vi "HTTP_Post.vi"(4 "data":string, 5 "URL":string="http://localhost:8086/api/v2/write?org=hassiosp&bucket=hassiosp&precision=ns", 6 "error in (no error)":errorcluster, 7 "value 3":string="application/json", 8 "value 2":string="text/plain; charset=utf-8", 9 "value 1":string="Token hassiosp") -> (0 "error out":errorcluster, 2 "body":string, 3 "headers":string)   [LabVIEW 2023]
uses:
  <vilib>/httpClient/POSTBuffer.vi
  <vilib>/httpClient/LabVIEWHTTPClient.lvlib
panel:
  in  "header 3":string(combo)="User-Agent"
  in  "header 2":string(combo)="Content-Type"
  in  "header 1":string="Authorization"
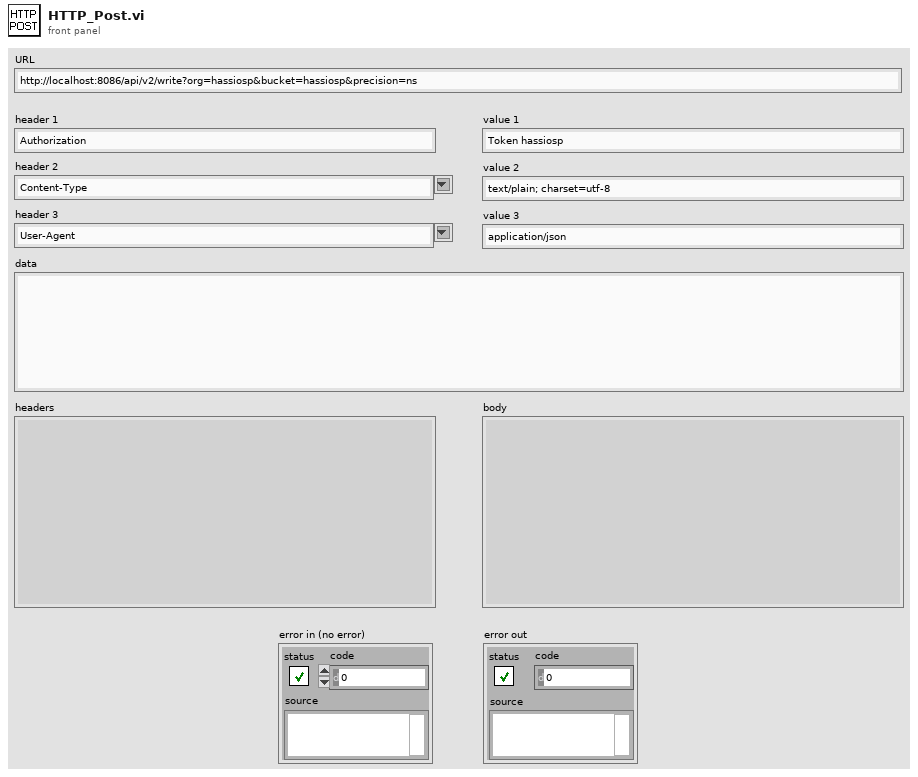
[diagram p1: front panel]
types:
  T1 = typedef "LabVIEWHTTPClient.lvlib/ClientHandle.ctl" = refnum<k1>
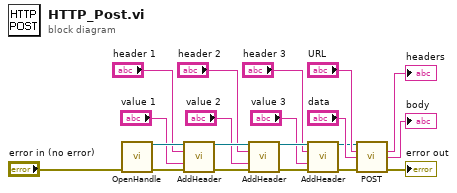
[diagram p0: block diagram]
diagram:
  n1 = call <vilib>:"OpenHandle.vi"("error in (no error)"="error in (no error)") -> ("client handle out"=w14:T1, "error out"=w13:errorcluster)  [unwired: 13 in]
  n2 = call <vilib>:"AddHeader.vi"("client handle"=w14, "header"="header 1", "value"="value 1", "error in (no error)"=w13) -> ("client handle out"=w15:T1, "error out"=w16:errorcluster)  [unwired: 10 in]
  n3 = call <vilib>:"AddHeader.vi"("client handle"=w15, "header"="header 2", "value"="value 2", "error in (no error)"=w16) -> ("client handle out"=w12:T1, "error out"=w11:errorcluster)  [unwired: 10 in]
  n4 = call <vilib>:"AddHeader.vi"("client handle"=w12, "header"="header 3", "value"="value 3", "error in (no error)"=w11) -> ("client handle out"=w9:T1, "error out"=w10:errorcluster)  [unwired: 10 in]
  n5 = call-poly <vilib>:"POST.vi"("client handle"=w9, "url"="URL", "buffer"="data", "error in (no error)"=w10) -> ("headers"=→"headers":string, "body"=→"body":string, "error out"=→"error out":errorcluster)  [unwired: 8 in, 1 out]
